vi "Persist Entities.vi"(8 "error in (no error)":errorcluster, 10 "Entities":refnum<class "Entity.lvclass">[](array[class]), 11 "SQLite in":refnum<class "SQLite.lvclass">) -> (0 "error out":errorcluster, 3 "SQLite out":refnum<class "SQLite.lvclass">)   [LabVIEW 2020, in "Conditum SQLite.lvlib" / "SQLite.lvclass"]
uses:
  SQLite.lvclass
  <vilib>/IlluminatedG/IG Conditum/Conditum/Entity/Entity.lvclass
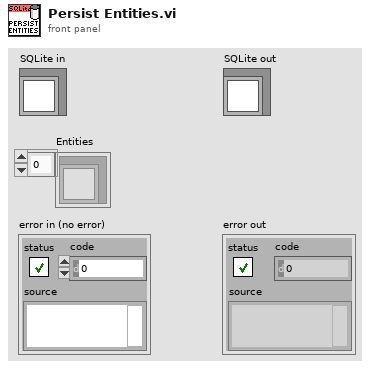
[diagram p1: front panel]
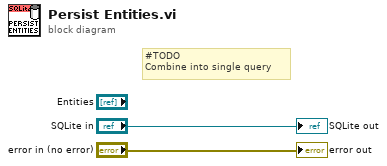
[diagram p0: block diagram]
diagram:
  # "#TODO\nCombine into single query"
  "error out" <- "error in (no error)"
  "SQLite out" <- "SQLite in"
